vi "CLStimSimple.vi"() -> ()   [LabVIEW 2017]
uses:
  <vilib>/DAQmx/write.llb/DAQmx Write (Analog Wfm 1Chan NSamp).vi
  <vilib>/DAQmx/read.llb/DAQmx Read (Counter U32 1Chan 1Samp).vi
  TTLReceive.vi
  <vilib>/DAQmx/miscellaneous.llb/DAQmx Fill In Error Info.vi
  <vilib>/addons/zeromq/zmq_recv_multi.vi
panel:
  in  "Sham stim channel":tag="pciDAQ/ao2"
  in  "Max add'l timeout (ms)":dbl=200.0
  in  "Sample rate":dbl=30000.0
  in  "Artifact length (ms)":dbl=1000.0
  in  "OEP sample clock in":tag="/pciDAQ/PFI0"
  in  "Onboard counter":tag="pciDAQ/ctr0"
  in  "Real stim channel":tag="pciDAQ/ao0"
  out "Learning rate (for adaptive threshold)":dbl(graph)
  out "Phase threshold":sgl(graph)
  in  "Sham stimulations:":i32=1 min=0
  in  "Real stimulations:":i32=1 min=1
  out "Stim time":i64
  out "Crossing time":i64
  out "Crossing level":sgl
  out "Time on (samp.)":i64
  in  "Sham TTL chan":u16=3 caption="probe channel" min=1 max=8
  in  "Crossing TTL chan":u16=1 min=1 max=8
  in  "event port":u16=5557
  out "New event":bool
  in  "Stim enabled":bool
  out "OEP to LV delay":dbl(graph)
  in  "Stop":bool
  # "*** Start OpenEphys acquisition before the VI. ***"
  # "*** In the audio settings in the OpenEphys GUI, reduce the buffer size to get a 10 ms buffer period.  If ASIO is installed and enabled in\nthe Open Ephys build, use ASIO with sample rate (in audio settings) = 192,000 Hz and buffer size = 192 (1 ms buffer period). ***"
  # "Inputs"
  # "Event info"
  # "Timeout"
  # "Stim pattern if enabled"
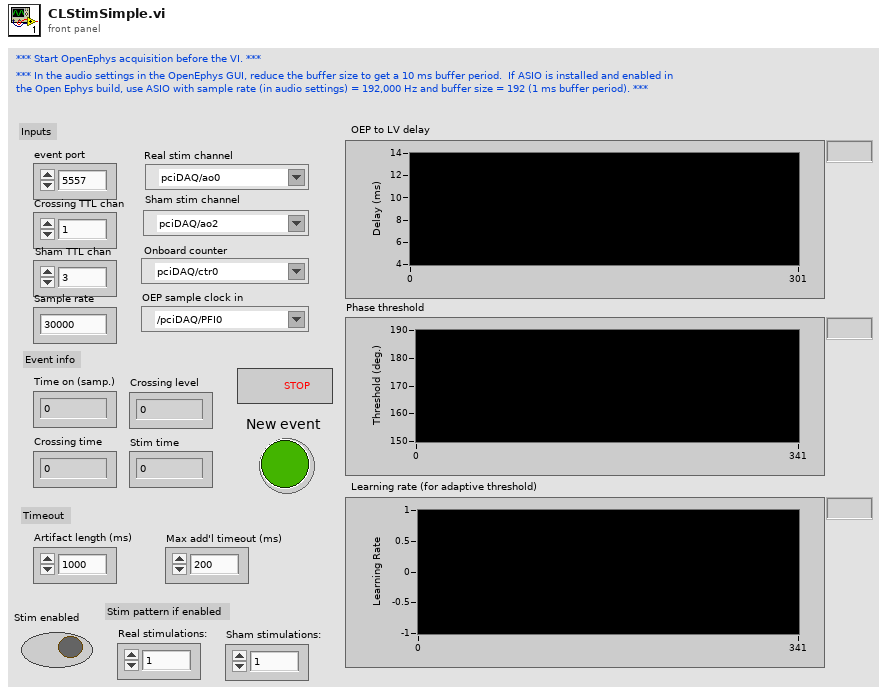
[diagram p1: front panel]
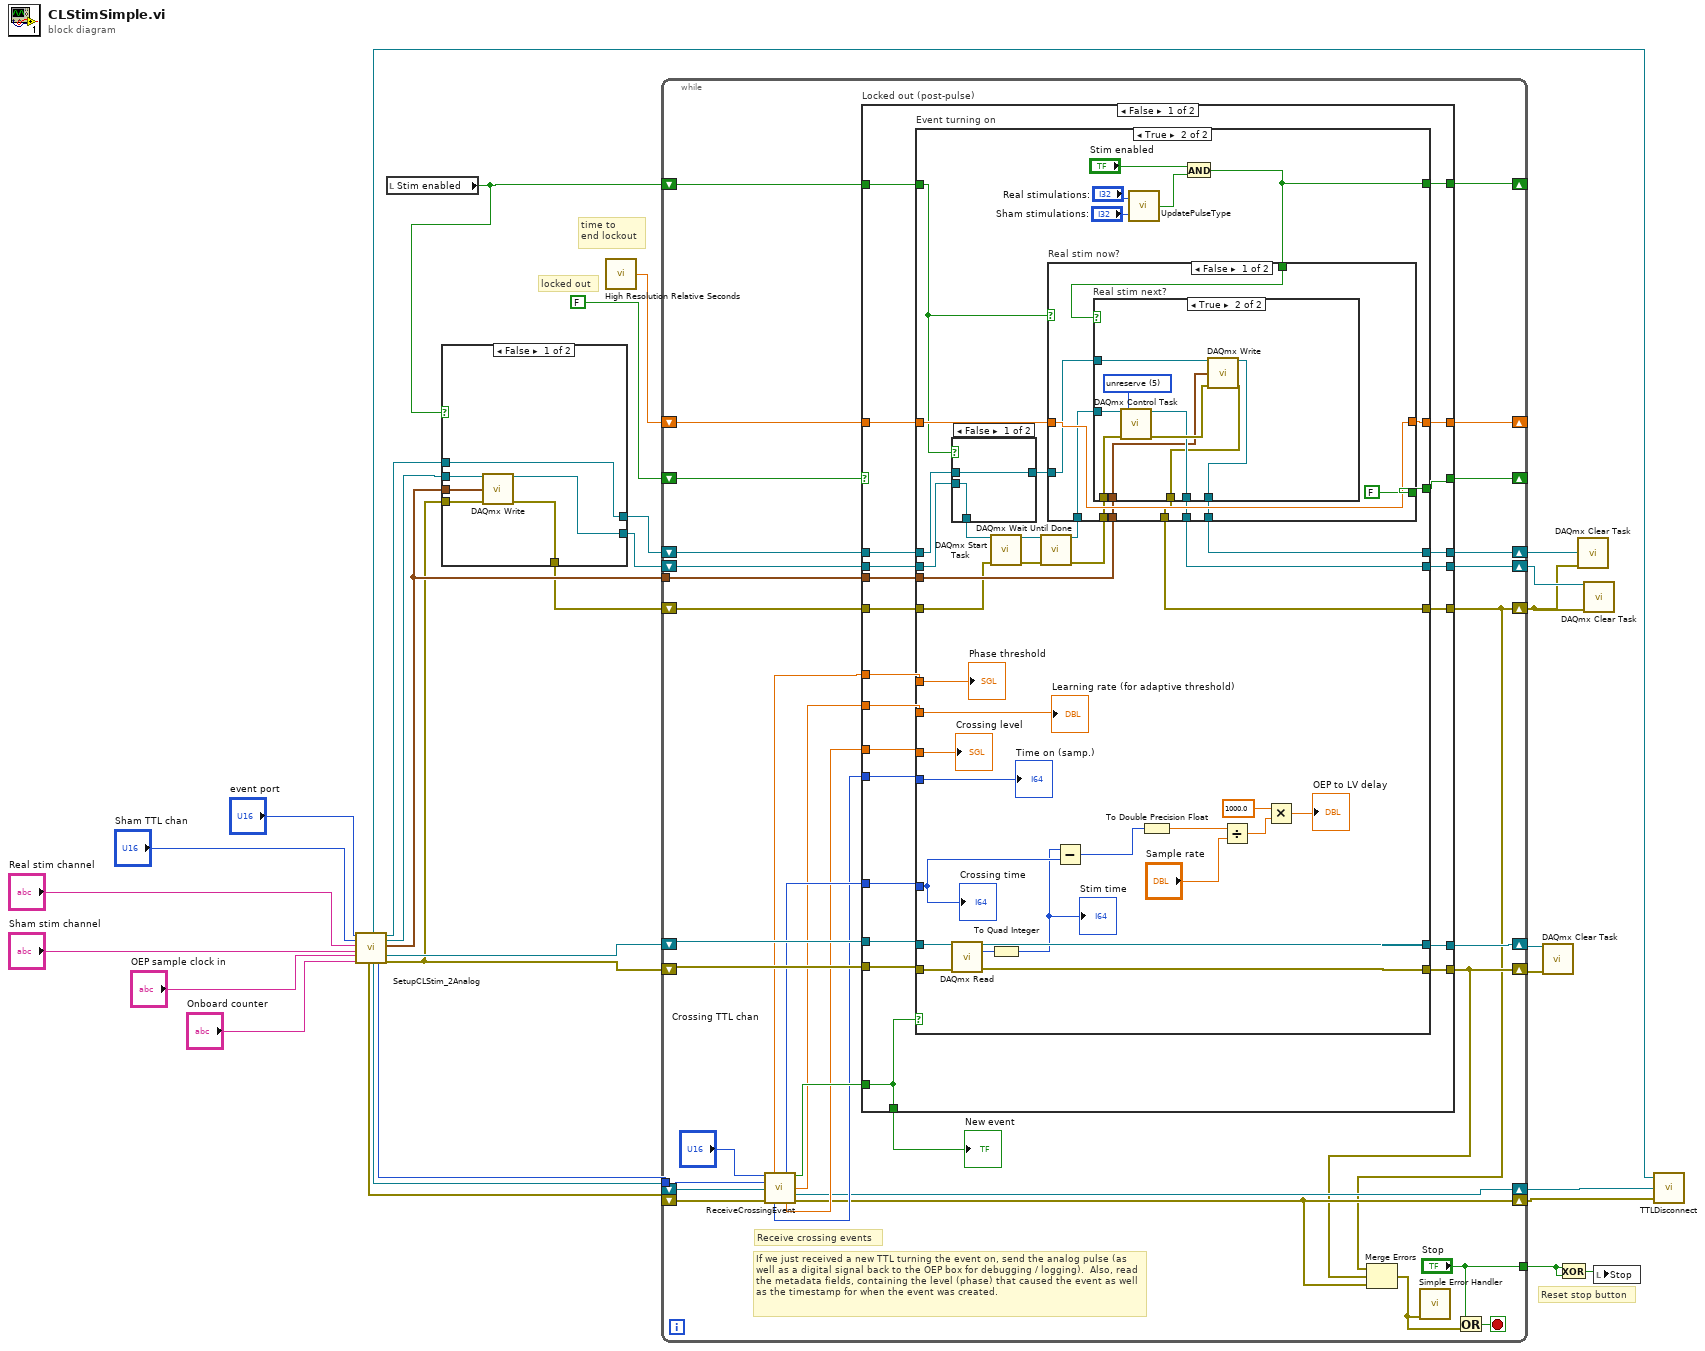
[diagram p0: block diagram]
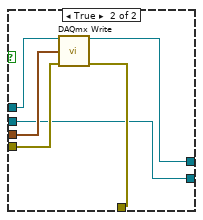
[diagram p2: hidden frame]
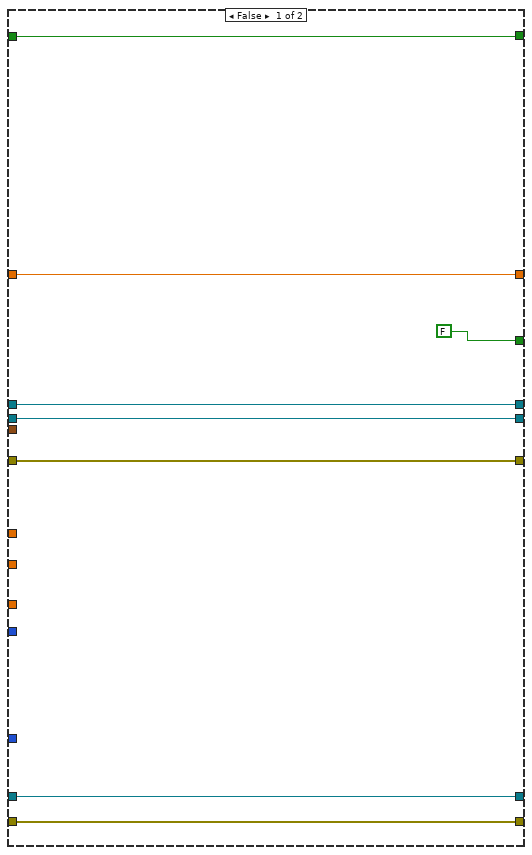
[diagram p3: hidden frame]
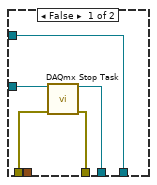
[diagram p5: hidden frame]
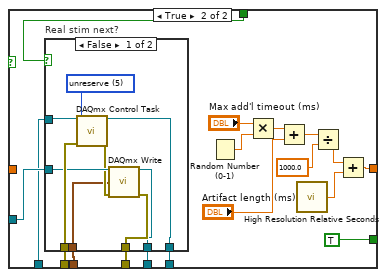
[diagram p6: hidden frame]
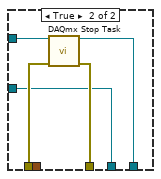
[diagram p7: hidden frame]
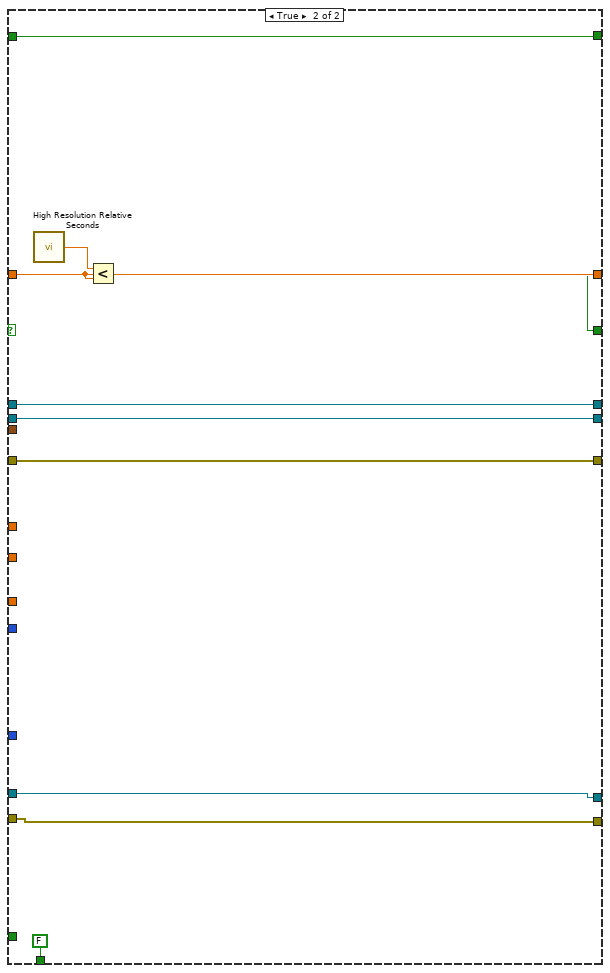
[diagram p8: hidden frame]
diagram:
  # "locked out"
  # "time to \nend lockout"
  # "Reset stop button"
  n1 = call "SetupCLStim_2Analog.vi"("event port"="event port", "Sham stim event channel"="Sham TTL chan", "Real stim channel"="Real stim channel", "Sham stim channel"="Sham stim channel", "OEP sample clock in"="OEP sample clock in", "Onboard counter"="Onboard counter") -> ("ZMQ error out"=w21:errorcluster, "context out"=w20:refnum<class "zmq_context.lvclass">, "socket out"=w22:refnum<class "zmq_socket.lvclass">, "clock offset"=w23:i64, "Real stim task"=w7:refnum<k21>, "Sham stim task"=w8:refnum<k21>, "Waveform Graph"=w6:waveform(dbl), "Ctr task"=w24:refnum<k21>, "DAQ error out"=w4:errorcluster)  [unwired: 5 in]
  n2 = local read "Stim enabled"() -> (w5:bool)
  n3 = case shown="False" w5 {
    tunnel: w8 -> [w34 w37]
    tunnel: w7 -> [w32 w41]
    tunnel: w6 -> [w35 w42]
    tunnel: w4 -> [w36 w40]
    tunnel: [w31 w39] -> w3
    tunnel: [w32 w38] -> w2
    tunnel: [w33 w37] -> w1
    frame False {
      n4 = call-poly <vilib>:"DAQmx Write.vi"("task/channels in"=w34, "data"=w35, "error in"=w36) -> ("task out"=w33:refnum<k21>, "error out"=w31:errorcluster)  [unwired: 10 in, 1 out]
    }
    frame True {
      n5 = call-poly <vilib>:"DAQmx Write.vi"("task/channels in"=w41, "data"=w42, "error in"=w40) -> ("task out"=w38:refnum<k21>, "error out"=w39:errorcluster)  [unwired: 10 in, 1 out]
    }
  }
  n6 = call <vilib>:"High Resolution Relative Seconds.vi"() -> ("relative seconds"=w16:dbl)
  n7 = while {
    tunnel: ["Stop"] -> w25
    shift-right: [w60] -> w11
    shift-left: w2 -> [w75]
    shift-right: [w45] -> w9
    shift-left: w3 -> [w73]
    shift-right: [w59] -> w29
    shift-left: w24 -> [w74]
    shift-right: [w55] -> w28
    shift-left: w4 -> [w72]
    shift-right: [w57] -> w27
    shift-left: w22 -> [w71]
    shift-right: [w56] -> w26
    shift-left: w21 -> [w70]
    tunnel: w23 -> [w54]
    shift-right: [w50] -> _
    shift-left: w16 -> [w49]
    shift-right: [w51] -> _
    shift-left: FALSE -> [w52]
    shift-right: [w47] -> w10
    shift-left: w1 -> [w48]
    tunnel: w6 -> [w46]
    shift-right: [w44] -> _
    shift-left: w5 -> [w43]
    stop <- w62 stop-if-true
    # "If we just received a new TTL turning the event on, send the analog pulse (as well as a digital signal back to the OEP box for debugging / logging).  Also, read the metadata fields, containing the level (phase) that caused the event as well as the timestamp for when the event was created."
    # "Receive crossing events"
    n8 = call "ReceiveCrossingEvent.vi"("channel"="Crossing TTL chan", "clock offset"=w54, "socket in"=w71, "error in"=w70) -> ("threshold"=w64:sgl, "new crossing"=w69:bool, "crossing time"=w68:i64, "learning rate"=w63:dbl, "socket out"=w57:refnum<class "zmq_socket.lvclass">, "event time"=w67:i64, "crossing level"=w66:sgl, "error out"=w56:errorcluster)  [unwired: 3 in, 1 out]
    n9 = case "Locked out (post-pulse)" shown="False" w52 {
      tunnel: w75 -> [w97 w211]
      tunnel: w74 -> [w96 w212]
      tunnel: w73 -> [w95 w210]
      tunnel: w72 -> [w94 w213]
      tunnel: w69 -> [w84 _]
      tunnel: w68 -> [w93 _]
      tunnel: w67 -> [w92 _]
      tunnel: w66 -> [w91 _]
      tunnel: w64 -> [w90 _]
      tunnel: w63 -> [w89 _]
      tunnel: [w88 w211] -> w60
      tunnel: [w87 w212] -> w59
      tunnel: [w86 w210] -> w45
      tunnel: [w85 w213] -> w55
      tunnel: [w84 FALSE ("new crossing")] -> w53
      tunnel: [w82 w207] -> w51
      tunnel: [w81 w209] -> w50
      tunnel: w49 -> [w83 w209]
      tunnel: w48 -> [w80 w206]
      tunnel: [w79 w206] -> w47
      tunnel: w46 -> [w78 _]
      tunnel: [w77 w205] -> w44
      tunnel: w43 -> [w76 w205]
      frame False {
        n10 = case "Event turning on" shown="True" w84 {
          tunnel: w97 -> [w105 w116]
          tunnel: w95 -> [w104 w119]
          tunnel: [w105 w110] -> w88
          tunnel: [w104 w109] -> w86
          tunnel: w93 -> [_ w138]
          tunnel: w96 -> [w103 w144]
          tunnel: w94 -> [w102 w142]
          tunnel: [w103 w141] -> w87
          tunnel: [w102 w140] -> w85
          tunnel: w92 -> [_ w139]
          tunnel: w91 -> [_ w137]
          tunnel: w90 -> [_ w136]
          tunnel: w89 -> [_ w135]
          tunnel: [w101 w124] -> w81
          tunnel: w83 -> [w101 w125]
          tunnel: [FALSE w123] -> w82
          tunnel: w80 -> [w99 w115]
          tunnel: [w99 w108] -> w79
          tunnel: w78 -> [_ w120]
          tunnel: [w98 w107] -> w77
          tunnel: w76 -> [w98 w106]
          frame False {
          }
          frame True {
            n11 = case shown="False" w106 {
              tunnel: w116 -> [w145 w148]
              tunnel: w115 -> [w146 w147]
              tunnel: [w146 w148] -> w114
              tunnel: [w145 w147] -> w113
              frame False {
              }
              frame True {
              }
            }
            n12 = call-poly <vilib>:"DAQmx Read.vi"("task/channels in"=w144, "error in"=w142) -> ("task out"=w141:refnum<k21>, "data"=w143:u32, "error out"=w140:errorcluster)  [unwired: 11 in]
            n13 = call <vilib>:"DAQmx Start Task.vi"("task/channels in"=w114, "error in"=w119) -> ("task out"=w118:refnum<k21>, "error out"=w117:errorcluster)  [unwired: 12 in]
            n14 = To Quad Integer(1:w143) -> (0:w134:i64)
            "Stim time" <- w134
            n15 = call <vilib>:"DAQmx Wait Until Done.vi"("task/channels in"=w118, "error in"=w117) -> ("task out"=w112:refnum<k21>, "error out"=w111:errorcluster)  [unwired: 12 in]
            n16 = Subtract(x=w134, y=w138) -> (x-y=w129:i64)
            n17 = call "UpdatePulseType.vi"("Sham stimulations:"="Sham stimulations:", "Real stimulations:"="Real stimulations:") -> ("Real stim on"=w121:bool)
            n18 = To Double Precision Float(number=w129) -> (double precision float=w131:dbl)
            n19 = And(x="Stim enabled", y=w121) -> (x .and. y?=w107:bool)
            n20 = case "Real stim now?" shown="False" w106 {
              tunnel: w125 -> [w158 _]
              tunnel: [w158 w190] -> w124
              tunnel: [FALSE TRUE] -> w123
              tunnel: w107 -> [w156 w180]
              tunnel: w120 -> [w149 w179]
              tunnel: w113 -> [w155 w178]
              tunnel: w112 -> [w154 w177]
              tunnel: w111 -> [w153 w176]
              tunnel: [w150 w175] -> w110
              tunnel: [w152 w174] -> w109
              tunnel: [w151 w173] -> w108
              frame False {
                n21 = case "Real stim next?" shown="True" w156 {
                  tunnel: w155 -> [w159 w167]
                  tunnel: w154 -> [w163 w172]
                  tunnel: w153 -> [w162 w171]
                  tunnel: [w161 w166] -> w152
                  tunnel: [w160 w168] -> w151
                  tunnel: [w159 w165] -> w150
                  tunnel: w149 -> [_ w164]
                  frame False {
                    n22 = call <vilib>:"DAQmx Stop Task.vi"("task/channels in"=w163, "error in"=w162) -> ("task out"=w160:refnum<k21>, "error out"=w161:errorcluster)  [unwired: 12 in]
                  }
                  frame True {
                    w170 = 5 items=["verify"=2, "reserve"=4, "commit"=3, "unreserve"=5, "abort"=6] ("action")
                    n23 = call <vilib>:"DAQmx Control Task.vi"("task/channels in"=w172, "action"=w170, "error in"=w171) -> ("task out"=w168:refnum<k21>, "error out"=w169:errorcluster)  [unwired: 11 in]
                    n24 = call-poly <vilib>:"DAQmx Write.vi"("task/channels in"=w167, "data"=w164, "error in"=w169) -> ("task out"=w165:refnum<k21>, "error out"=w166:errorcluster)  [unwired: 10 in, 1 out]
                  }
                }
              }
              frame True {
                n25 = case "Real stim next?" shown="False" w180 {
                  tunnel: w179 -> [w194 _]
                  tunnel: w178 -> [w196 w201]
                  tunnel: w177 -> [w199 w204]
                  tunnel: w176 -> [w197 w203]
                  tunnel: [w193 w200] -> w175
                  tunnel: [w192 w202] -> w174
                  tunnel: [w191 w201] -> w173
                  frame False {
                    w198 = 5 items=["verify"=2, "reserve"=4, "commit"=3, "unreserve"=5, "abort"=6] ("action")
                    n26 = call <vilib>:"DAQmx Control Task.vi"("task/channels in"=w199, "action"=w198, "error in"=w197) -> ("task out"=w193:refnum<k21>, "error out"=w195:errorcluster)  [unwired: 11 in]
                    n27 = call-poly <vilib>:"DAQmx Write.vi"("task/channels in"=w196, "data"=w194, "error in"=w195) -> ("task out"=w191:refnum<k21>, "error out"=w192:errorcluster)  [unwired: 10 in, 1 out]
                  }
                  frame True {
                    n28 = call <vilib>:"DAQmx Stop Task.vi"("task/channels in"=w204, "error in"=w203) -> ("task out"=w200:refnum<k21>, "error out"=w202:errorcluster)  [unwired: 12 in]
                  }
                }
                n29 = Random Number (0-1)() -> (number: 0 to 1=w188:dbl)
                n30 = Multiply(x="Max add'l timeout (ms)", y=w188) -> (x*y=w183:dbl)
                n31 = Add(x=w183, y="Artifact length (ms)") -> (x+y=w185:dbl)
                n32 = call <vilib>:"High Resolution Relative Seconds.vi"() -> ("relative seconds"=w181:dbl)
                n33 = Divide(x=w185, y=1000.0) -> (x/y=w186:dbl)
                n34 = Add(x=w186, y=w181) -> (x+y=w190:dbl)
              }
            }
            n35 = Divide(x=w131, y="Sample rate") -> (x/y=w127:dbl)
            n36 = Multiply(x=1000.0, y=w127) -> (x*y=→"OEP to LV delay":dbl)
            "Time on (samp.)" <- w139
            "Crossing time" <- w138
            "Crossing level" <- w137
            "Phase threshold" <- w136
            "Learning rate (for adaptive threshold)" <- w135
          }
        }
      }
      frame True {
        n37 = call <vilib>:"High Resolution Relative Seconds.vi"() -> ("relative seconds"=w208:dbl)
        n38 = Less?(x=w208, y=w209) -> (x < y?=w207:bool)
      }
    }
    "New event" <- w53
    n39 = Merge Errors(w45, w55, w56) -> (w58:errorcluster)
    n40 = call <vilib>:"Simple Error Handler.vi"("error in (no error)"=w58) -> ()  [unwired: 4 in, 5 out]
    n41 = Or(x="Stop", y=w58) -> (x .or. y?=w62:bool)
  }
  n42 = call <vilib>:"DAQmx Clear Task.vi"("task in"=w29, "error in"=w28) -> ()  [unwired: 13 in, 1 out]
  n43 = Exclusive Or(1:w25, 2:w25) -> (0:w30:bool)
  n44 = call <vilib>:"DAQmx Clear Task.vi"("task in"=w11, "error in"=w9) -> ()  [unwired: 13 in, 1 out]
  n45 = call <vilib>:"DAQmx Clear Task.vi"("task in"=w10, "error in"=w9) -> ()  [unwired: 13 in, 1 out]
  n46 = local write "Stop"(w30) -> ()
  n47 = call "TTLDisconnect.vi"("error in"=w26, "socket in"=w27, "context in"=w20) -> ()  [unwired: 1 in, 1 out]
